vi "PH_PowerUnit_BaseClass.get PU Tagname.vi"(1 "PU Tag":T2, 2 "PU":T1) -> (0 "PU Tagname":string)   [LabVIEW 2014, in "PH_PowerUnit_BaseClass.lvlib"]
doc: "This VI concatenates a Tagname out of strict type def enum controls. It keeps also the information whether the Tag is existing (if not, N/A is given out as name)."
uses:
  PH_PowerUnit_BaseClass.lvlib
  PH_PowerUnit_BaseClass.PP PU Tags.ctl
  PH_PP_Common/PH_PP_Common.PUs.ctl
  PH_PP_Common/PH_PP_Common.Devices.ctl
  PH_Common/Names/PH_Names.Subsystems.ctl
  PH_Common/Names/PH_Names.Communication Type.ctl
  PH_Common/PH_Common.lvlib
  PH_PP_Common/PH_PP_Common.lvlib
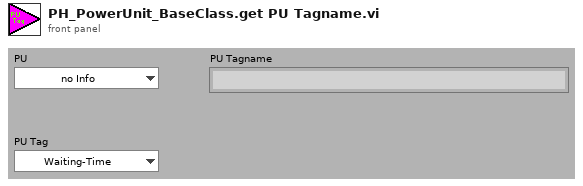
[diagram p1: front panel]
types:
  T1 = typedef "PH_PP_Common.lvlib/PH_PP_Common.PUs.ctl" = enum16{"no Info", "PA-19mm-1", "PA-19mm-2", "PA-45mm-PILC", "PA-45mm-MAIN", "MA-PU-1", "MA-PU-2", "MA-PU-3", "MA-PU-4", "MA-PU-5", "MA-PU-6", "MA-FR", "MA-PILC", "PA-45mm-DP"}
  T2 = typedef "PH_PowerUnit_BaseClass.lvlib/PH_PowerUnit_BaseClass.PP PU Tags.ctl" = enum16{"Waiting-Time", "PU-in-Use"}
  T3 = typedef "PH_Common.lvlib/PH_Names.Communication Type.ctl" = enum16{"no Info", "SE", "SA", "AE", "AA", "DE", "DA", "DIM"}
  T4 = typedef "PH_Common.lvlib/PH_Names.Subsystems.ctl" = enum16{"no Info", "fs-FE", "ns-FE", "PA", "MA", "MAS", "COS", "Exp-LB", "Exp-LL", "PP", "PILS"}
  T5 = typedef "PH_PP_Common.lvlib/PH_PP_Common.Devices.ctl" = enum16{"no Info", "Igni", "RR", "DumpRoss", "PSU", "Trigger", "HV-Meas", "Rods", "Chiller", "Conductivity", "Mercury"}
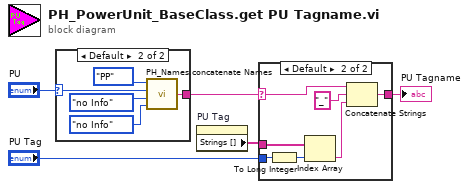
[diagram p0: block diagram]
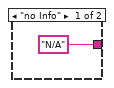
[diagram p2: hidden frame]
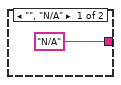
[diagram p3: hidden frame]
diagram:
  n1 = case shown="Default" "PU" {
    selector: "PU" -> [_ w10]
    tunnel: ["N/A" ("Subsystem_PU_Devices_Comm Type") w11] -> w4
    frame "no Info" {
    }
    frame Default {
      n2 = call "PH_Names.concatenate Names.vi"("Communication Type (no info)"=PH_Names.Communication_Type."no Info", "Devices (no info)"=PH_PP_Common.Devices."no Info", "PU (no info)"=w10, "Subsystem"=PH_Names.Subsystems."PP") -> ("Subsystem_PU_Devices_Comm Type"=w11:string)
    }
  }
  n3 = property on="PU Tag" class="Enum (strict)"() -> ("Strings []"=w3:string[])  [unwired: 2 in, 2 out]
  n4 = case shown="Default" w4 {
    selector: w4 -> [_ w13]
    tunnel: ["N/A" w19] -> w5
    tunnel: w3 -> [_ w18]
    tunnel: "PU Tag" -> [_ w14]
    frame "", "N/A" {
    }
    frame Default {
      n5 = To Long Integer(number=w14) -> (32bit integer=w17:i32)
      n6 = Index Array(array=w18, index=w17) -> (element=w16:string)
      n7 = Concatenate Strings(w13, "_" ("string"), w16) -> (w19:string)
    }
  }
  "PU Tagname" <- w5
